vi "Highlight Write.vi"(4 "error in (no error)":errorcluster, 5 "Value":i32, 6 "Container State":T6, 7 "Display State In":T1={"Nspeakers"=13, "actions"=[], "Wspeaker"=13, "hover"={"type"=enum."None", "index"=0}, "locked"=FALSE, "states"=[], "sel speak"=13, "selected"=refnum, "Events"={"Selection change"=refnum}}) -> (0 "error out":errorcluster, 3 "Display State Out":T1={"Nspeakers"=13, "actions"=[], "Wspeaker"=13, "hover"={"type"=enum."None", "index"=0}, "locked"=FALSE, "states"=[], "sel speak"=13, "selected"=refnum, "Events"={"Selection change"=refnum}})   [LabVIEW 2015, in "SAC Config.xctl"]
uses:
  SAC Config.xctl
  <vilib>/_xctls/Container State.ctl
  State.vi
  Hover Data.ctl
  Hover Item.ctl
  Speaker State.ctl
  Events.ctl
  Selection changed.ctl
  <vilib>/_xctls/XControlSupport.lvlib
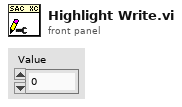
[diagram p1: front panel]
types:
  T1 = typedef "SAC Config.xctl/State.vi" = cluster{"Nspeakers":i32, "actions":string[], "Wspeaker":i32, "hover":T2, "locked":bool, "states":T4[], "sel speak":i32, "selected":refnum<vi>, "Events":T5}
  T2 = typedef "SAC Config.xctl/Hover Data.ctl" = cluster{"type":T3, "index":i32}
  T3 = typedef "SAC Config.xctl/Hover Item.ctl" = enum16{"None", "Speaker"}
  T4 = typedef "SAC Config.xctl/Speaker State.ctl" = cluster{"cal":bool, "selected":bool}
  T5 = typedef "SAC Config.xctl/Events.ctl" = cluster{"Selection change":refnum<user-event>}
  T6 = typedef "XControlSupport.lvlib/Container State.ctl" = cluster{"Indicator?":bool, "Run Mode?":bool, " Refnum":refnum<vi>}
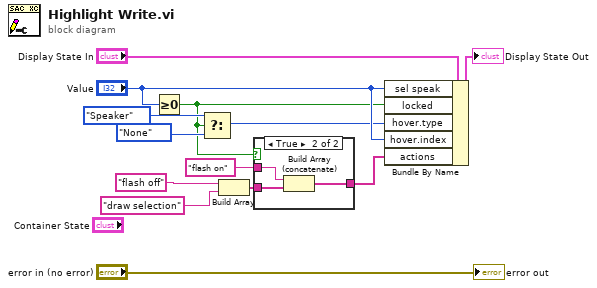
[diagram p0: block diagram]
diagram:
  n1 = Greater Or Equal To 0?(x="Value") -> (x >= 0?=w3:bool)
  n2 = Select(t=Hover_Item."Speaker", s=w3, f=Hover_Item."None" ("hover.type")) -> (s? t:f=w8:T3)
  n3 = Build Array("flash off" ("action"), "draw selection" ("action")) -> (w4:string[])
  n4 = case shown="True" w3 {
    tunnel: w4 -> [w14 w17]
    tunnel: "flash on" ("action") -> [_ w16]
    tunnel: [w14 w15] -> w1
    frame False {
    }
    frame True {
      n5 = Build Array (concatenate)(w16, w17) -> (w15:string[])
    }
  }
  n6 = Bundle By Name(cluster="Display State In", "sel speak"="Value", "locked"=w3, "hover.type"=w8, "hover.index"="Value", "actions"=w1) -> (→"Display State Out":T1)
  "error out" <- "error in (no error)"
